vi "Calcolo_Distanza.vi"(0 "Ingresso in MicroSecondi":string) -> (1 "Metri":dbl, 2 "Centimetri":dbl)   [LabVIEW 2018]
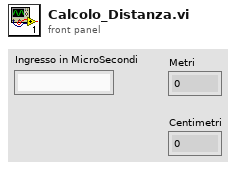
[diagram p1: front panel]
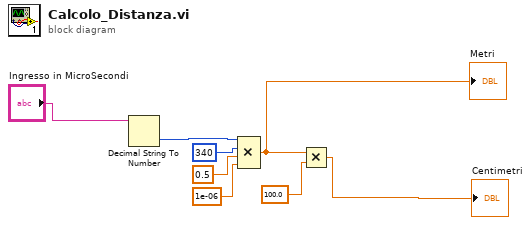
[diagram p0: block diagram]
diagram:
  n1 = Decimal String To Number(string="Ingresso in MicroSecondi") -> (number=w2:i32)  [unwired: 2 in, 1 out]
  n2 = Compound Arithmetic op=MULTIPLY(w2, 340, 0.5, 1e-06) -> (w4:dbl)
  "Metri" <- w4
  n3 = Multiply(x=w4, y=100.0) -> (x*y=→"Centimetri":dbl)
